vi "Route Start Trigger.vi"(6 "trigger master index":i32, 8 "error in (no error)":errorcluster, 10 "start trigger rtsi line":string, 11 "fpga interfaces in":refnum<k20>[](array[refnum])) -> (0 "error out":errorcluster, 3 "fpga interfaces out":refnum<k20>[](array[refnum]))   [LabVIEW 2021]
uses:
  <instrlib>/FlexRIO/API/Host/v1/NI FlexRIO/API/Configure Digital Edge Start Trigger.vi
  <instrlib>/FlexRIO/API/Host/v1/NI FlexRIO/API/Get Property Reference - Fpga Small.vi
  <instrlib>/FlexRIO/API/Host/v1/NI FlexRIO API v1.lvlib
  <resource>/objmgr/sessionReference.rc
  <resource>/objmgr/niflexrioapi.rc
  <resource>/objmgr/niflexrioapiTrigger.rc
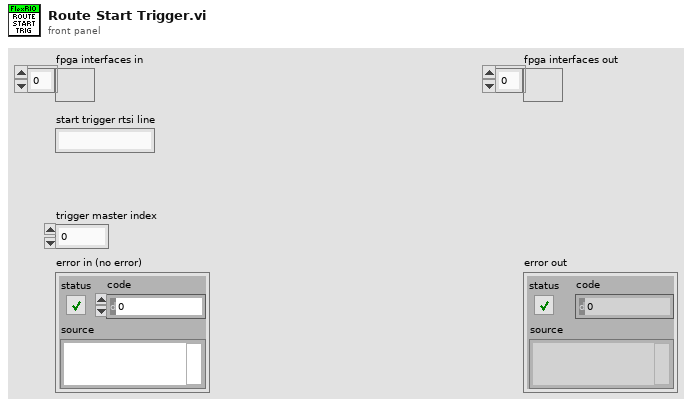
[diagram p1: front panel]
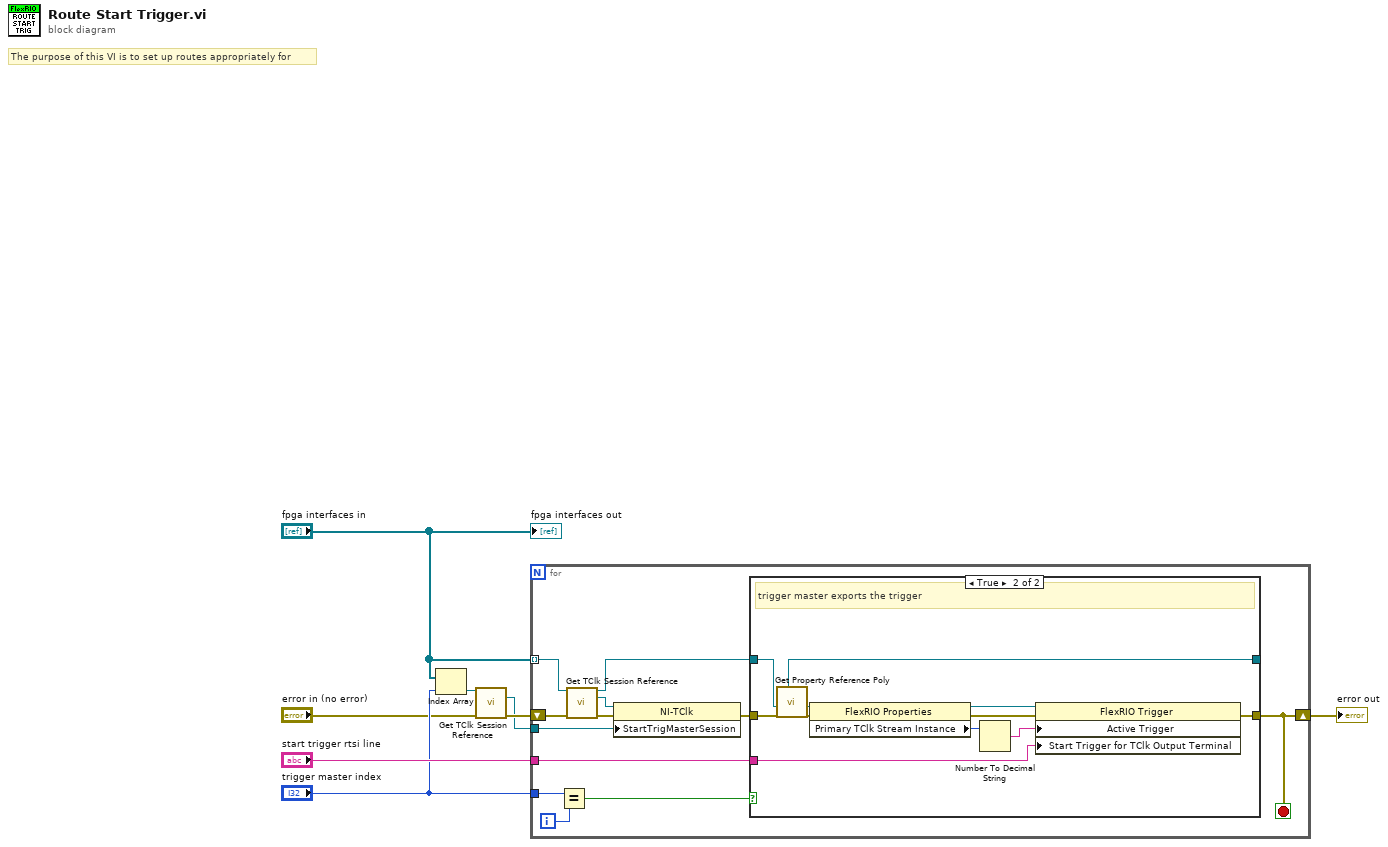
[diagram p0: block diagram]
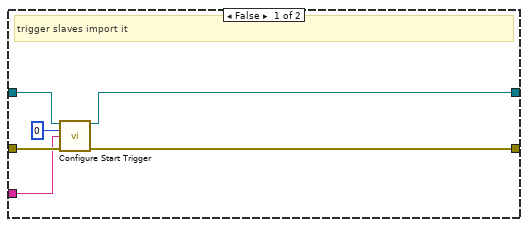
[diagram p2: hidden frame]
diagram:
  # "The purpose of this VI is to set up routes appropriately for"
  n1 = Index Array(array="fpga interfaces in", index="trigger master index") -> (element=w5:refnum<k20>)
  n2 = call <instrlib>:"Get TClk Session Reference.vi"("fpga interface in"=w5, "error in"="error in (no error)") -> ("tclk session reference"=w4:refnum<k20>, "error out"=w6:errorcluster)  [unwired: 11 in, 1 out]
  n3 = for {
    tunnel: "start trigger rtsi line" -> [w11]
    shift-right: [w9] -> w2
    shift-left: w6 -> [w18]
    tunnel: "trigger master index" -> [w20]
    tunnel: "fpga interfaces in" -> [w19] mode=indexing
    tunnel: w4 -> [w17]
    i -> [w10]
    stop <- w9 stop-if-true
    n4 = Equal?(x=w20, y=w10) -> (x = y?=w14:bool)
    n5 = call <instrlib>:"Get TClk Session Reference.vi"("fpga interface in"=w19, "error in"=w18) -> ("fpga interface out"=w12:refnum<k20>, "tclk session reference"=w15:refnum<k20>, "error out"=w16:errorcluster)  [unwired: 11 in]
    n6 = property class="NI-TClk"(reference=w15, error in=w16, "StartTrigMasterSession"=w17) -> (error out=w13:errorcluster)  [unwired: 1 out]
    n7 = case shown="True" w14 {
      tunnel: w13 -> [w26 w34]
      tunnel: w12 -> [w24 w35]
      tunnel: w11 -> [w23 w32]
      tunnel: [w22 w27] -> _
      tunnel: [w21 w28] -> w9
      frame False {
        # "trigger slaves import it"
        n8 = call-poly <instrlib>:"Configure Start Trigger.vi"("fpga interface in"=w24, "trigger instance"=u32 0, "trigger source"=w23, "error in"=w26) -> ("fpga interface out"=w22:refnum<k20>, "error out"=w21:errorcluster)  [unwired: 9 in, 1 out]
      }
      frame True {
        # "trigger master exports the trigger"
        n9 = call-poly <instrlib>:"Get Property Reference Poly.vi"("error in (no error)"=w34, "fpga interface in"=w35) -> ("error out"=w36:errorcluster, "property reference"=w37:refnum<k20>, "fpga interface out"=w27:refnum<k20>)  [unwired: 4 in]
        n10 = property class="FlexRIO Properties"(reference=w37, error in=w36) -> (reference out=w31:refnum<k20>, error out=w33:errorcluster, "Primary TClk Stream Instance"=w30:i32)
        n11 = Number To Decimal String(number=w30) -> (decimal integer string=w29:string)  [unwired: 1 in]
        n12 = property class="FlexRIO Trigger"(reference=w31, error in=w33, "Active Trigger"=w29, "Start Trigger for TClk Output Terminal"=w32) -> (error out=w28:errorcluster)  [unwired: 1 out]
      }
    }
  }
  "error out" <- w2
  "fpga interfaces out" <- "fpga interfaces in"
